vi "Sub_predictor(SubVI).vi"(7 "Sim_running":bool, 8 "outer":dbl, 9 "middle":dbl, 10 "inner":dbl, 11 "t [s]":dbl) -> (1 "outer vec":dbl[](array[numeric]), 2 "middle vec":dbl[](array[numeric]), 3 "inner vec":dbl[](array[numeric]))   [LabVIEW 2017]
uses:
  <vilib>/Analysis/_algsub.llb/Real PseudoInverse Matrix.vi
  <vilib>/Analysis/baseanly.llb/Real A x B.vi
  <vilib>/Analysis/Matrix/Numeric/Conversions/Array To Matrix - RA.vi
  <vilib>/Analysis/Matrix/Numeric/Conversions/Array To Matrix - RA2.vi
  <vilib>/Analysis/Matrix/Numeric/Conversions/Matrix To Array - RM.vi
  <vilib>/Analysis/Matrix/NI_Matrix.lvlib
  <vilib>/Analysis/NI_AALPro.lvlib
  <vilib>/Analysis/NI_AALBase.lvlib
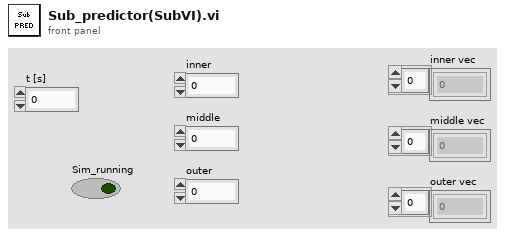
[diagram p1: front panel]
types:
  T1 = typedef "NI_Matrix.lvlib/RealMatrix.ctl" = dbl[][]
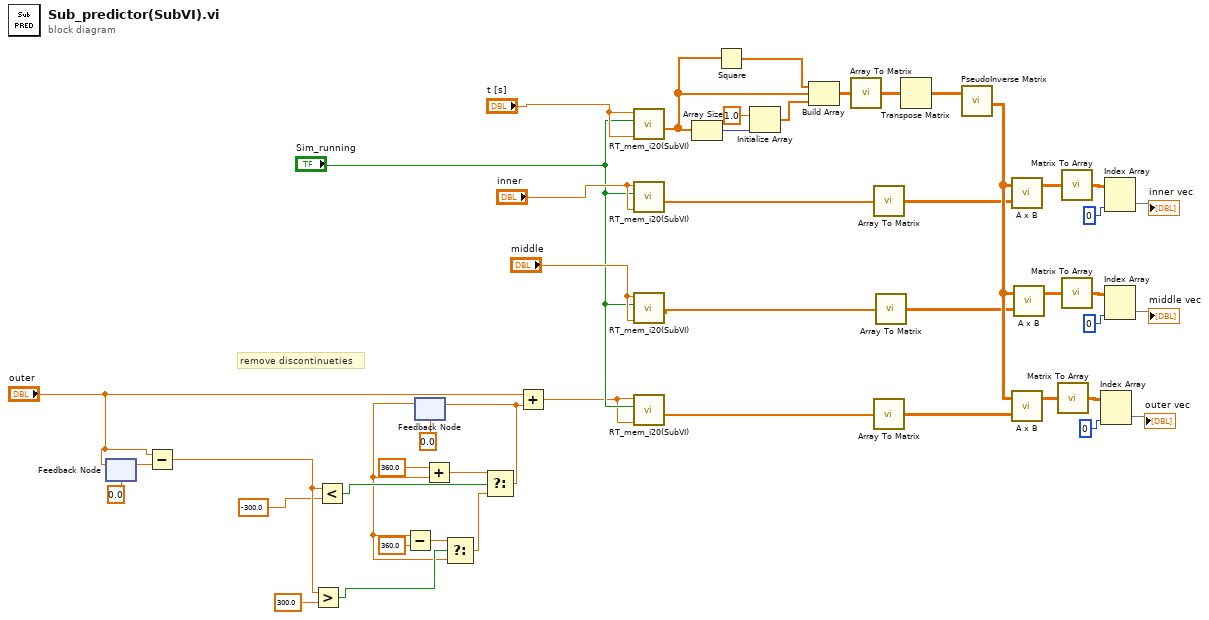
[diagram p0: block diagram]
diagram:
  # "remove discontinueties"
  n1 = feedback #1(0.0 ("outer")) -> (w4:dbl)
  n2 = feedback-in #1("outer") -> ()
  n3 = Subtract(x="outer", y=w4) -> (x-y=w3:dbl)
  n4 = Greater?(x=w3, y=300.0) -> (0:w14:bool)
  n5 = Less?(x=w3, y=-300.0) -> (x < y?=w16:bool)
  n6 = feedback #2(0.0) -> (w10:dbl)
  n7 = Subtract(x=w10, y=360.0) -> (x-y=w13:dbl)
  n8 = Add(x=360.0, y=w10) -> (x+y=w11:dbl)
  n9 = Select(t=w13, s=w14, f=w10) -> (s? t:f=w12:dbl)
  n10 = Select(t=w11, s=w16, f=w12) -> (s? t:f=w6:dbl)
  n11 = feedback-in #2(w6) -> ()
  n12 = Add(x="outer", y=w6) -> (x+y=w17:dbl)
  n13 = call "RT_mem_i20(SubVI).vi"("Ini_val"="t [s]", "start"="Sim_running", "In"="t [s]") -> ("in_vec"=w21:dbl[])  [unwired: 7 in, 1 out]
  n14 = call "RT_mem_i20(SubVI).vi"("Ini_val"="inner", "start"="Sim_running", "In"="inner") -> ("in_vec"=w35:dbl[])  [unwired: 7 in, 1 out]
  n15 = call "RT_mem_i20(SubVI).vi"("Ini_val"="middle", "start"="Sim_running", "In"="middle") -> ("in_vec"=w31:dbl[])  [unwired: 7 in, 1 out]
  n16 = call "RT_mem_i20(SubVI).vi"("Ini_val"=w17, "start"="Sim_running", "In"=w17) -> ("in_vec"=w36:dbl[])  [unwired: 7 in, 1 out]
  n17 = Array Size(array=w21) -> (size(s)=w18:i32)
  n18 = Square(x=w21) -> (x^2=w20:dbl[])
  n19 = Initialize Array(1.0 ("element"), w18) -> (w22:dbl[])
  n20 = Build Array(w20, w21, w22) -> (w24:dbl[][])
  n21 = call-poly <vilib>:"Array To Matrix.vi"("Real 2D Array"=w24) -> ("Real Matrix"=w23:T1)
  n22 = call-poly <vilib>:"Array To Matrix.vi"("Real 1D Array"=w35) -> ("Real Matrix (Column Vector)"=w33:T1)
  n23 = call-poly <vilib>:"Array To Matrix.vi"("Real 1D Array"=w36) -> ("Real Matrix (Column Vector)"=w34:T1)
  n24 = call-poly <vilib>:"Array To Matrix.vi"("Real 1D Array"=w31) -> ("Real Matrix (Column Vector)"=w26:T1)
  n25 = Transpose Matrix(1:w23) -> (0:w25:T1)
  n26 = call-poly <vilib>:"PseudoInverse Matrix.vi"("Input Matrix"=w25) -> ("PseudoInverse Matrix"=w43:T1)  [unwired: 1 in, 1 out]
  n27 = call-poly <vilib>:"A x B.vi"("B"=w33, "A"=w43) -> ("A x B"=w44:T1)  [unwired: 1 out]
  n28 = call-poly <vilib>:"A x B.vi"("B"=w34, "A"=w43) -> ("A x B"=w45:T1)  [unwired: 1 out]
  n29 = call-poly <vilib>:"A x B.vi"("B"=w26, "A"=w43) -> ("A x B"=w29:T1)  [unwired: 1 out]
  n30 = call-poly <vilib>:"Matrix To Array.vi"("Real Matrix"=w45) -> ("Real 2D Array"=w40:dbl[][])
  n31 = call-poly <vilib>:"Matrix To Array.vi"("Real Matrix"=w44) -> ("Real 2D Array"=w39:dbl[][])
  n32 = call-poly <vilib>:"Matrix To Array.vi"("Real Matrix"=w29) -> ("Real 2D Array"=w27:dbl[][])
  n33 = Index Array(array=w40, index (col)=0 ("index (row)")) -> (element=→"outer vec":dbl[])  [unwired: 1 in]
  n34 = Index Array(array=w39, index (col)=0 ("index (row)")) -> (element=→"inner vec":dbl[])  [unwired: 1 in]
  n35 = Index Array(array=w27, index (col)=0 ("index (row)")) -> (element=→"middle vec":dbl[])  [unwired: 1 in]
